vi "Create_Tag.vi"(8 "error in (no error)":errorcluster, 10 "timeout":i32=1000, 11 "PLC Attributes":T1={"protocol"="ab_eip", "path"="1,0", "gatewayIP"="192.168.1.40", "cpu"="LGX", "element size"="", "element count"="1", "tag name"="din_LCEDiveVC", "debug level"="NONE"}) -> (0 "error out":errorcluster, 2 "error code":i32, 3 "handle":i32=28)   [LabVIEW 2019]
uses:
  PLC_Attributes.ctl
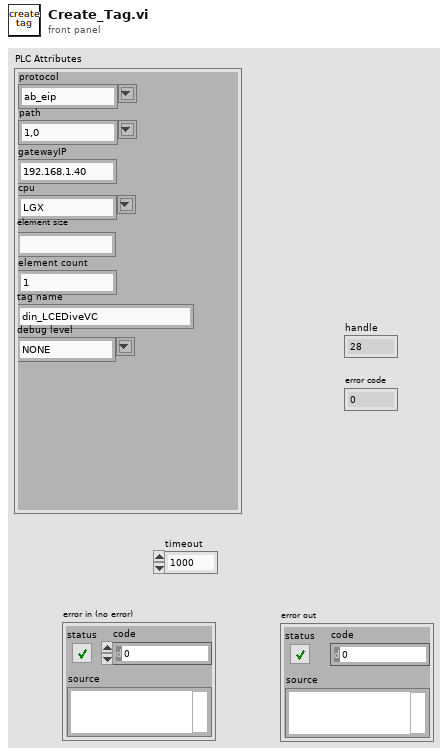
[diagram p1: front panel]
types:
  T1 = typedef "PLC_Attributes.ctl" = cluster{"protocol":string, "path":string, "gatewayIP":string, "cpu":string, "element size":string, "element count":string, "tag name":string, "debug level":string}
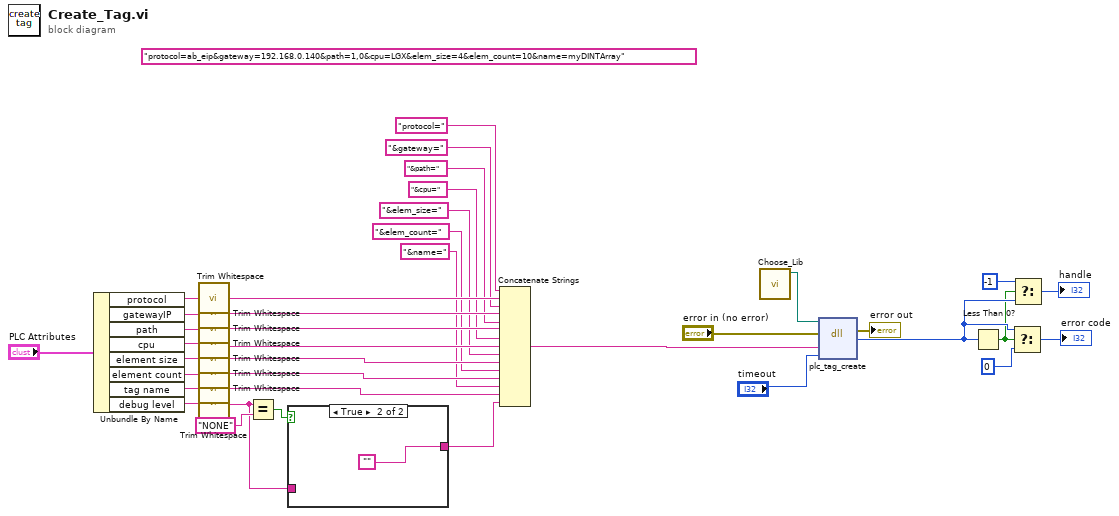
[diagram p0: block diagram]
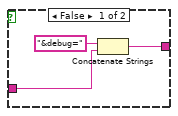
[diagram p2: hidden frame]
diagram:
  (unwired) "protocol=ab_eip&gateway=192.168.0.140&path=1,0&cpu=LGX&elem_size=4&elem_count=10&name=myDINTArray"
  n1 = Unbundle By Name("PLC Attributes") -> ("protocol"=w31:string, "gatewayIP"=w30:string, "path"=w29:string, "cpu"=w28:string, "element size"=w26:string, "element count"=w27:string, "tag name"=w25:string, "debug level"=w24:string)
  n2 = call <vilib>:"Trim Whitespace.vi"("string"=w31) -> ("trimmed string"=w22:string)  [unwired: 1 in]
  n3 = call <vilib>:"Trim Whitespace.vi"("string"=w30) -> ("trimmed string"=w20:string)  [unwired: 1 in]
  n4 = call <vilib>:"Trim Whitespace.vi"("string"=w29) -> ("trimmed string"=w18:string)  [unwired: 1 in]
  n5 = call <vilib>:"Trim Whitespace.vi"("string"=w28) -> ("trimmed string"=w16:string)  [unwired: 1 in]
  n6 = call <vilib>:"Trim Whitespace.vi"("string"=w26) -> ("trimmed string"=w14:string)  [unwired: 1 in]
  n7 = call <vilib>:"Trim Whitespace.vi"("string"=w27) -> ("trimmed string"=w12:string)  [unwired: 1 in]
  n8 = call <vilib>:"Trim Whitespace.vi"("string"=w25) -> ("trimmed string"=w10:string)  [unwired: 1 in]
  n9 = call <vilib>:"Trim Whitespace.vi"("string"=w24) -> ("trimmed string"=w7:string)  [unwired: 1 in]
  n10 = Equal?(x=w7, y="NONE") -> (x = y?=w8:bool)
  n11 = case shown="True" w8 {
    tunnel: w7 -> [w40 _]
    tunnel: [w39 ""] -> w6
    frame False {
      n12 = Concatenate Strings("&debug=", w40) -> (w39:string)
    }
    frame True {
    }
  }
  n13 = Concatenate Strings("protocol=", w22, "&gateway=", w20, "&path=", w18, "&cpu=", w16, "&elem_size=", w14, "&elem_count=", w12, "&name=", w10, w6) -> (w5:string)
  n14 = call "Choose_Lib.vi"() -> ("appended path"=w1:path)  [unwired: 11 in]
  n15 = dll-call lib="?" fn="plc_tag_create"(path in=w1, error in="error in (no error)", "IP address"=w5, "timeout"="timeout") -> (error out=→"error out":errorcluster, "return type"=w35:i32)  [unwired: 3 in, 1 out]
  n16 = Less Than 0?(x=w35) -> (x < 0?=w34:bool)
  n17 = Select(t=w35, s=w34, f=0) -> (s? t:f=→"error code":i32)
  n18 = Select(t=-1, s=w34, f=w35) -> (s? t:f=→"handle":i32)
